vi "decimo.vi"() -> ()   [LabVIEW 2012]
panel:
  out "XY Graph":cluster{i32[], i32[]}(graph)
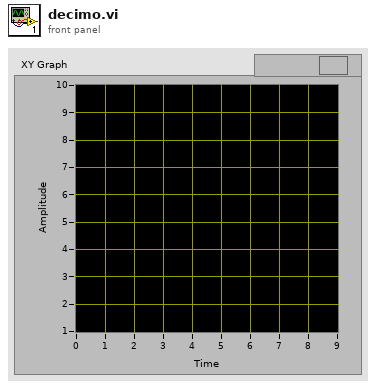
[diagram p1: front panel]
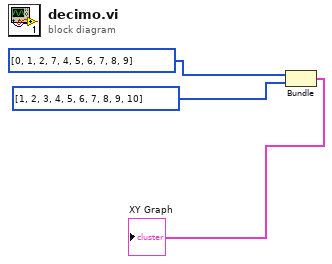
[diagram p0: block diagram]
diagram:
  n1 = Bundle(i32[] [0, 1, 2, 7, 4, 5, 6, 7, 8, 9], i32[] [1, 2, 3, 4, 5, 6, 7, 8, 9, 10]) -> (→"XY Graph":cluster{i32[], i32[]})  [unwired: 1 in]
